vi "WLAN - TV - RW - Refernce(RX).vi"() -> (2 "Rx Measurements Settings":T1[](array[typedef])=[{"Standard"=0, "Channel Bandwidth (Hz)"=20000000.0, "Idle Interval (s)"=0.0004, "MCS Index"=0, "80211n PLCP Frame Format"=0, "Payload Data Length (bytes)"=980, "OFDM Data Rate (Mbps)"=0, "DSSS Data Rate (Mbps)"=0, "Carrier Frequency(Hz)"=[2412000000.0, 2442000000.0, 2472000000.0, 5260000000.0, 5600000000.0, 5785000000.0], "Start Power Level(dBm)"=-10.0, "Stop Power Level(dBm)"=-100.0, "Step Size"=-1.0}, {"Standard"=1, "Channel Bandwidth (Hz)"=20000000.0, "Idle Interval (s)"=0.0004, "MCS Index"=0, "80211n PLCP Frame Format"=0, "Payload Data Length (bytes)"=200, "OFDM Data Rate (Mbps)"=0, "DSSS Data Rate (Mbps)"=0, "Carrier Frequency(Hz)"=[2412000000.0, 2442000000.0, 2472000000.0], "Start Power Level(dBm)"=-10.0, "Stop Power Level(dBm)"=-100.0, "Step Size"=-1.0}, {"Standard"=1, "Channel Bandwidth (Hz)"=20000000.0, "Idle Interval (s)"=0.0004, "MCS Index"=0, "80211n PLCP Frame Format"=0, "Payload Data Length (bytes)"=980, "OFDM Data Rate (Mbps)"=0, "DSSS Data Rate (Mbps)"=4, "Carrier Frequency(Hz)"=[2412000000.0, 2442000000.0, 2472000000.0], "Start Power Level(dBm)"=-10.0, "Stop Power Level(dBm)"=-100.0, "Step Size"=-1.0}, {"Standard"=3, "Channel Bandwidth (Hz)"=20000000.0, "Idle Interval (s)"=0.0004, "MCS Index"=0, "80211n PLCP Frame Format"=0, "Payload Data Length (bytes)"=980, "OFDM Data Rate (Mbps)"=0, "DSSS Data Rate (Mbps)"=0, "Carrier Frequency(Hz)"=[5260000000.0, 5600000000.0, 5785000000.0, 2412000000.0, 2442000000.0, 2472000000.0], "Start Power Level(dBm)"=-10.0, "Stop Power Level(dBm)"=-100.0, "Step Size"=-1.0}, {"Standard"=3, "Channel Bandwidth (Hz)"=20000000.0, "Idle Interval (s)"=0.0004, "MCS Index"=7, "80211n PLCP Frame Format"=0, "Payload Data Length (bytes)"=980, "OFDM Data Rate (Mbps)"=0, "DSSS Data Rate (Mbps)"=0, "Carrier Frequency(Hz)"=[2412000000.0, 2442000000.0, 2472000000.0, 5260000000.0, 5600000000.0, 5785000000.0], "Start Power Level(dBm)"=-10.0, "Stop Power Level(dBm)"=-100.0, "Step Size"=-1.0}, {"Standard"=3, "Channel Bandwidth (Hz)"=40000000.0, "Idle Interval (s)"=0.0004, "MCS Index"=0, "80211n PLCP Frame Format"=0, "Payload Data Length (bytes)"=1024, "OFDM Data Rate (Mbps)"=0, "DSSS Data Rate (Mbps)"=0, "Carrier Frequency(Hz)"=[5190000000.0, 5230000000.0, 5310000000.0, 5510000000.0, 5630000000.0, 5670000000.0, 5755000000.0, 5795000000.0], "Start Power Level(dBm)"=-10.0, "Stop Power Level(dBm)"=-100.0, "Step Size"=-1.0}, {"Standard"=3, "Channel Bandwidth (Hz)"=40000000.0, "Idle Interval (s)"=0.0004, "MCS Index"=7, "80211n PLCP Frame Format"=0, "Payload Data Length (bytes)"=1024, "OFDM Data Rate (Mbps)"=0, "DSSS Data Rate (Mbps)"=0, "Carrier Frequency(Hz)"=[5190000000.0, 5230000000.0, 5310000000.0, 5510000000.0, 5630000000.0, 5670000000.0, 5755000000.0, 5795000000.0], "Start Power Level(dBm)"=-10.0, "Stop Power Level(dBm)"=-100.0, "Step Size"=-1.0}] {"DSSS Data Rate (Mbps)" items=["1", "2", "5.5 CCK", "5.5 PBCC", "11 CCK", "11 PBCC", "22", "33"]; "OFDM Data Rate (Mbps)" items=["6", "9", "12", "18", "24", "36", "48", "54"]; "80211n PLCP Frame Format" items=["Mixed Format", "Greenfield Format"]; "Standard" items=["80211A/G/J/P OFDM", "80211B/G DSSS", "80211G DSSSOFDM", "80211N MIMOOFDM", "80211AC MIMOOFDM"]})   [LabVIEW 2011]
uses:
  Includes/WLAN - TV - RW - INC - TV_Rx_Measurements.ctl
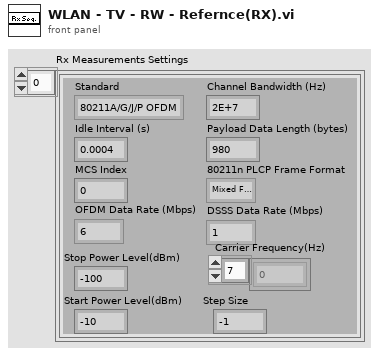
[diagram p1: front panel]
types:
  T1 = typedef "WLAN - TV - RW - INC - TV_Rx_Measurements.ctl" = cluster{"Standard":i32, "Channel Bandwidth (Hz)":dbl, "Idle Interval (s)":dbl, "MCS Index":i32, "80211n PLCP Frame Format":i32, "Payload Data Length (bytes)":i32, "OFDM Data Rate (Mbps)":i32, "DSSS Data Rate (Mbps)":i32, "Carrier Frequency(Hz)":dbl[], "Start Power Level(dBm)":dbl, "Stop Power Level(dBm)":dbl, "Step Size":dbl}
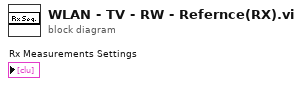
[diagram p0: block diagram]
diagram:
